vi "Dashboard Main.vi"() -> ()   [LabVIEW 2013]
uses:
  <vilib>/Rock Robotics/SystemInterfaces/AI/FPGA_AIChannel.ctl
  <vilib>/Rock Robotics/SystemInterfaces/Typedef/FPGA_TypedefAnalogModule.ctl
  <vilib>/event_ctls.llb/eventvkey.ctl
  <vilib>/Rock Robotics/WPI/Dashboard/WPI_DashboardLogging Global.vi
  <vilib>/Utility/config.llb/Write Key (String).vi
  <vilib>/Utility/config.llb/Write Key (I32).vi
  <vilib>/Utility/config.llb/NI_LVConfig.lvlib
panel:
  out "Image Message":string="Timeout in Camera Communications"
  in  "Dashboard Tab":T1(tab)
  in  "Camera Settings":T2={"Frame Rate"=30, "Compression"=30, "Size"=1} {"Frame Rate" scale=1.0..30.0; "Size" items=["640x480", "320x240", "160x120"]}
  out "MotorSliders R":cluster{"MotorSlide1":dbl, "MotorSlide2":dbl} {"MotorSlide2" scale=-1.0..1.0 scale format="%#_2e"; "MotorSlide1" scale=-1.0..1.0 scale format="%#_2e"}
  out "MotorChart R":cluster{"Numeric":dbl, "Numeric":dbl}(graph)
  out "MotorSliders L":T3 {"MotorSlide4 2" scale=0.0..14.0 scale format="%#_2e"; "MotorSlide2" scale=-1.0..1.0 scale format="%#_2e"; "MotorSlide1" scale=-1.0..1.0 scale format="%#_2e"}
  out "MotorChart L":T4(graph)
  out "JS1 Z":dbl(slide) scale=-1.0..1.0 scale format="%#_2e"
  out "Joystick 1":cluster{"X":dbl, "Y":dbl}[](graph)
  out "JS Buttons 1":T5
  out "JS2 Z":dbl(slide) scale=-1.0..1.0 scale format="%#_2e"
  out "Joystick 2":cluster{"X":dbl, "Y":dbl}[](graph)
  out "JS Buttons 2":T5
  out "Mode":T6(ring)=enum."Auto Disabled"
  out "Camera IP":string
  in  "DB Camera Config":bool
  out "fps":dbl format="%#.1g"
  out "Mbps":dbl format="%#.1g"
  out "Mbps 2":bool
  out "LED 1":bool
  in  "Enable":bool
  in  "?":dbl(slide) scale=0.0..100.0
  in  "Rec Mode":enum32{"Stop", "Record", "Playback"}(radio)
  out "distance":dbl(slide)=125.0 scale=0.0..250.0 scale format="%3d"
  in  "Scaling factor (V/in)":dbl=0.0098
  in  "Analog Module":T7
  in  "Samples Per Second":dbl=1000.0
  in  "Average Bits":u8=3 max=15
  in  "Channel":T8
  in  "stop":bool
  in  "Slider 1":dbl(slide) scale=0.0..100.0
  in  "Checkbox 2":bool
  in  "Checkbox 1":bool
  in  "Test Slider":dbl(slide) scale=0.0..100.0 scale format="%#_3g"
  in  "On/Off":bool caption="Solenoid"
  in  "Test Name":u16(ring) items=["Select the test to run...", "Example Test", "-------------------------------", "List of tests is built in robot code.", "Replace with your own automated tests."]
  in  "Test Tree":string(tree)
  in  "Motor":cluster{"Value":dbl, "Enable":bool} {"Value" scale=-1.0..1.0 scale format="%#_3g"}
  out "Progress":T9 {"Test Progress" scale=0.0..100.0}
  in  "Rev/Fwd":cluster{"Forward":bool, "Reverse":bool}
  in  "Test Ring":u16(ring) items=["Auto", "Fixed indoor", "Fixed outdoor 1", "Fixed outdoor 2", "Fixed fluorescent 1", "Fixed fluorescent 2", "Hold current"]
  in  "Listbox":i32(listbox)
  out "Tree":string(tree)
  out "Camera Image":T10(plugin-control)
  # "Left"
  # "Front"
  # "Right"
  # "Battery"
  # "Customize by placing controls and indicators here and name to\nmatch Dashboard Variables on robot."
  # "These can be set while running."
  # "Set these inputs before running."
  # "Output information."
  # "EZ1"
  # "inches"
  # "This tab is a great place for autonomous settings and validation.\nCustomize by placing controls and indicators here and name to\nmatch Dashboard Variables on robot."
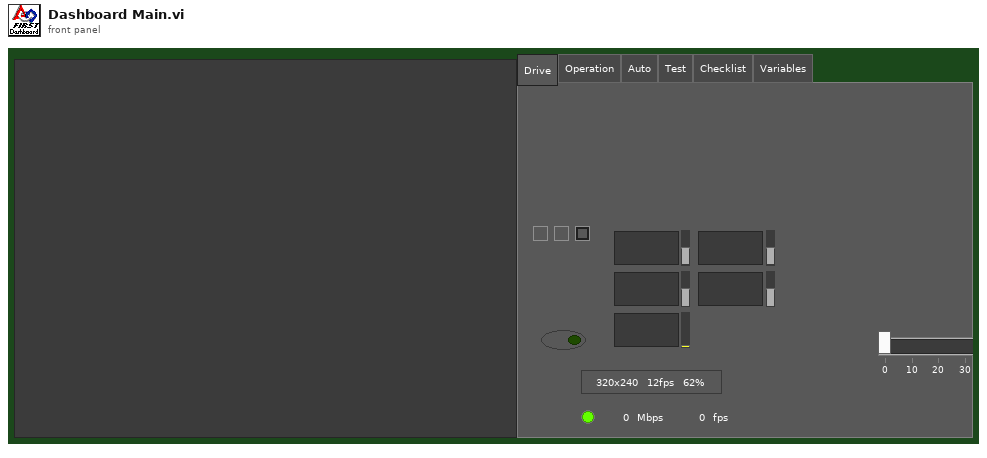
[diagram p1: front panel]
types:
  T1 = enum32{"Drive", "Operation", "Auto", "Test", "Checklist", "Variables"}
  T2 = cluster{"Frame Rate":i32, "Compression":i32, "Size":u16}
  T3 = cluster{"MotorSlide1":dbl, "MotorSlide2":dbl, "MotorSlide4 2":dbl}
  T4 = cluster{"Numeric":dbl, "Numeric":dbl, "Battery":sgl}
  T5 = cluster{bool, bool, bool, bool, bool, bool, bool, bool, bool, bool, bool, bool}
  T6 = enum8{"Tele-Op Disabled", "Tele-Op Enabled", "Auto Disabled", "Auto Enabled", "Test Disabled", "Test Enabled", ""}
  T7 = typedef "FPGA_TypedefAnalogModule.ctl" = enum16{"Analog Module 1", "Analog Module 2"}
  T8 = typedef "FPGA_AIChannel.ctl" = enum8{"AI 1", "AI 2", "AI 3", "AI 4", "AI 5", "AI 6", "AI 7", "AI 8", "Invalid"}
  T9 = cluster{"Test Progress":u8, "Test Progress Text":string}
  T10 = typedef "IMAQ Image.ctl" = refnum<image>
  T11 = typedef "Image Type" = u32
  T12 = cluster{"Digital Inputs":bool[], "Digital Outputs":bool[]}
  T13 = cluster{"Competition mode":bool, "Robot Link":bool, "Autonomous":bool, "Enabled":bool, "E-Stop":bool, "Simulated":bool, "TestMode":bool, "Docked Window":bool}
  T14 = cluster{"Boolean Array[0]":bool, "Boolean Array[1]":bool, "Boolean Array[2]":bool, "Boolean Array[3]":bool, "Boolean Array[4]":bool, "Boolean Array[5]":bool, "Boolean Array[6]":bool, "Boolean Array[7]":bool, "Boolean Array[8]":bool, "Boolean Array[9]":bool, "Boolean Array[10]":bool, "Boolean Array[11]":bool}
  T15 = typedef "NI_LVConfig.lvlib/Config Data RefNum.ctl" = refnum<k1>
  T16 = typedef "eventvkey.ctl" = enum16{"ASCII", "Enter", "Return", "Shift", "Ctrl", "Alt", "Cmd", "Opt", "Caps", "NumLock", "Clear", "Break", "Up", "Down", "Left", "Right", "Insert", "Delete", "Home", "End", "PageUp", "PageDown", "Escape", "Help", "Pause", "ScrollLock", "F1", "F2", "F3", "F4", "F5", "F6", "F7", "F8", "F9", "F10", "F11", "F12", "F13", "F14", "F15", "F16", "F17", "F18", "F19", "F20", "F21", "F22", "F23", "F24", "Play", "VolumeUp", "VolumeDown", "Mute", "Two Byte Char"}
  T17 = cluster{"Image Size":bool, "Image Type":bool, "Pixel Value":bool, "ROI Information":bool, "Zoom Factor":bool}
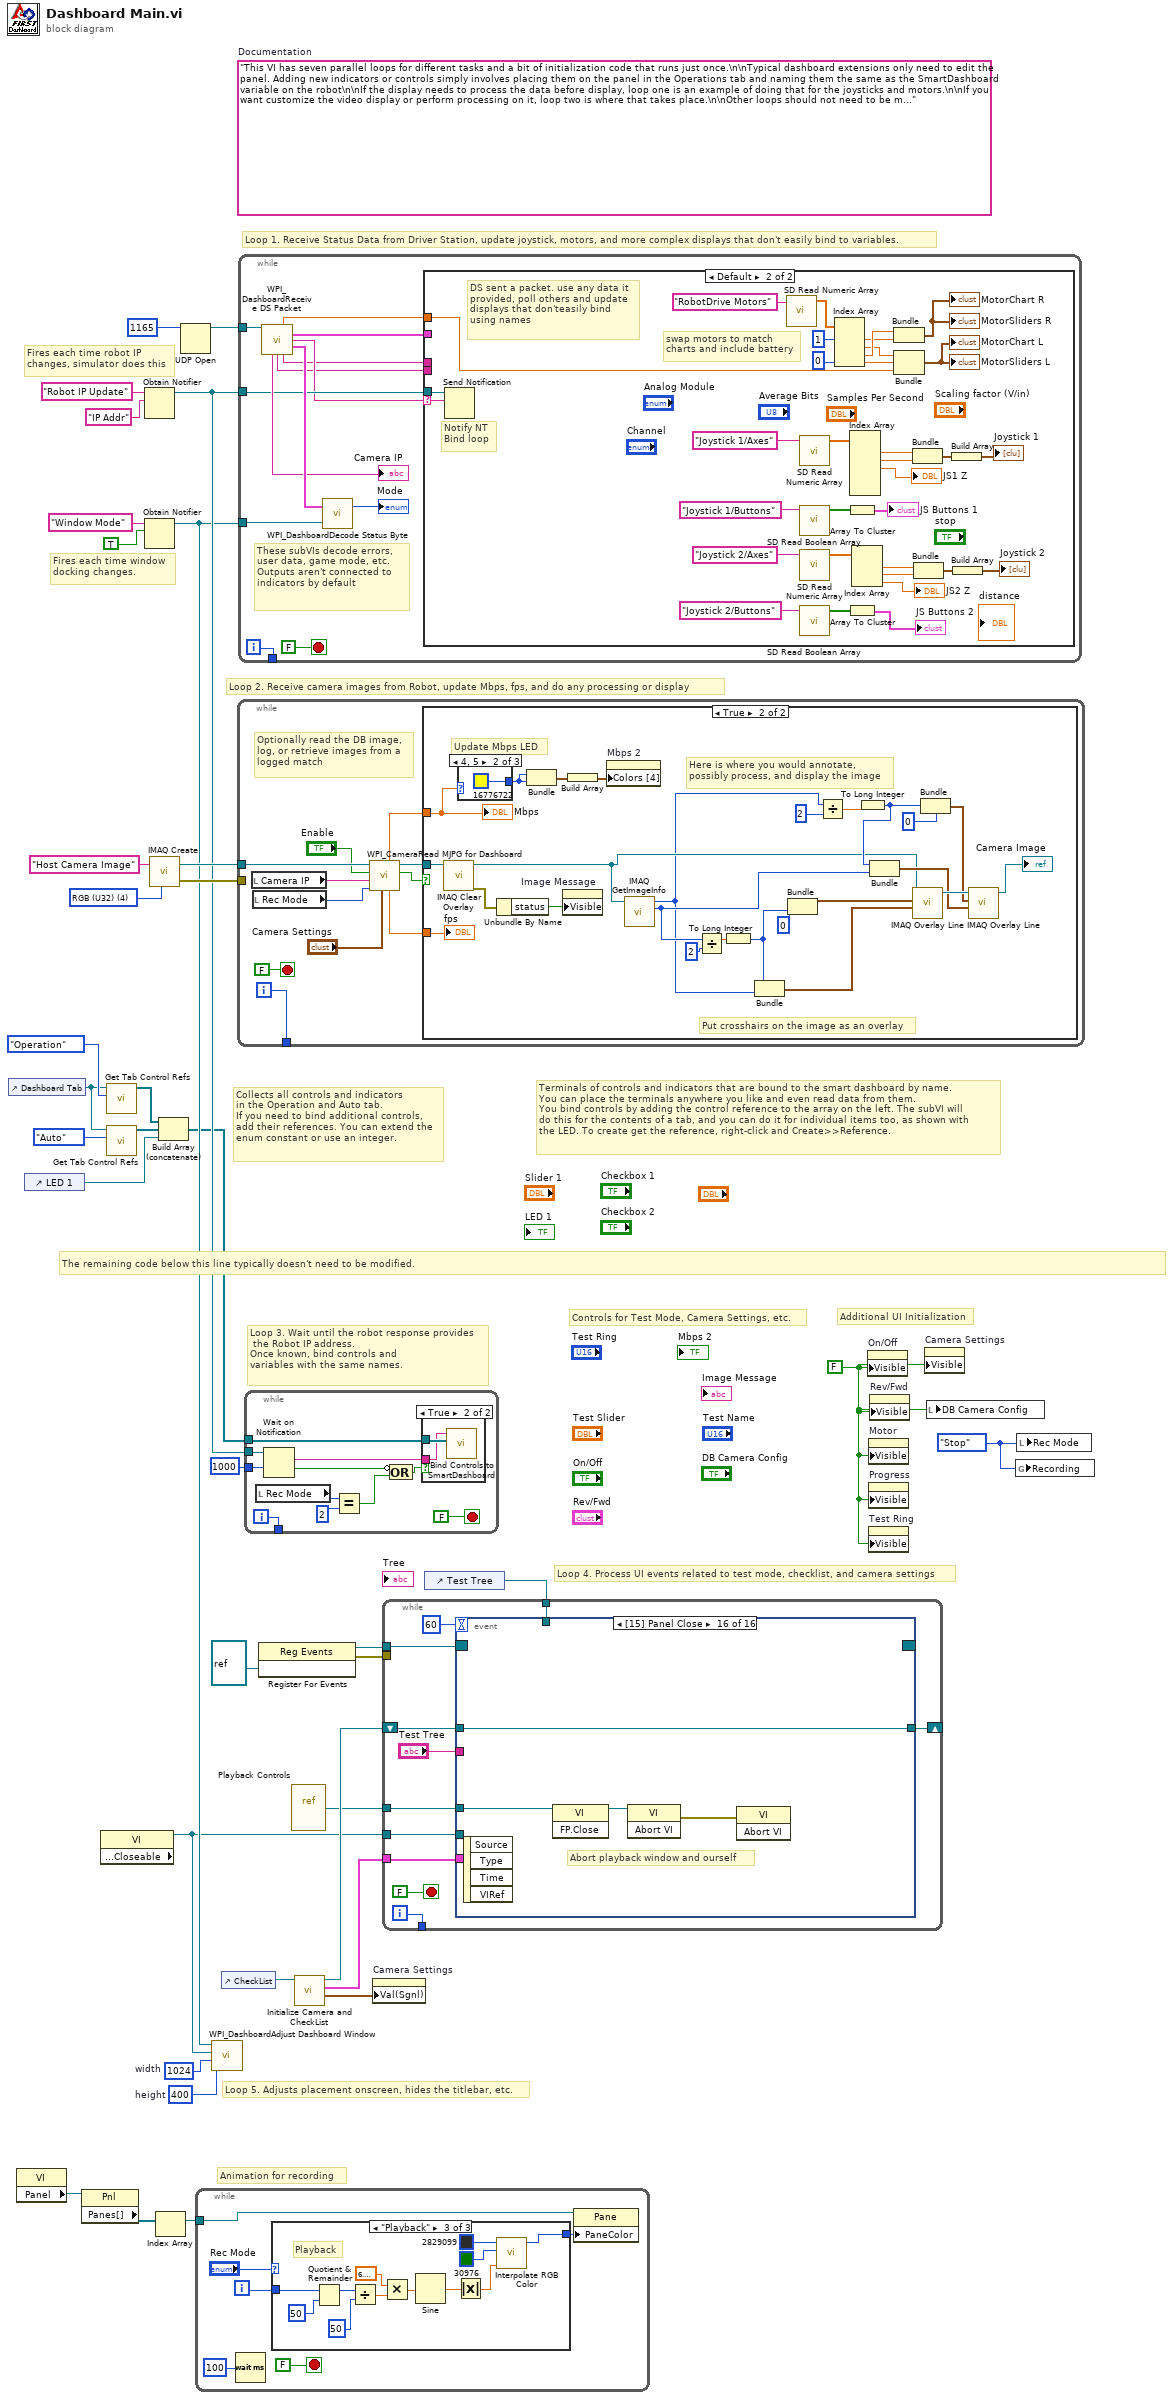
[diagram p0: block diagram]
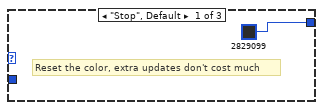
[diagram p2: hidden frame]
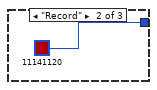
[diagram p3: hidden frame]
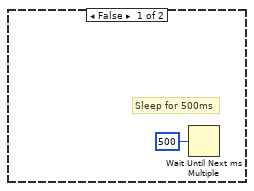
[diagram p5: hidden frame]
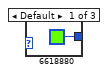
[diagram p6: hidden frame]
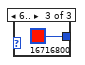
[diagram p7: hidden frame]
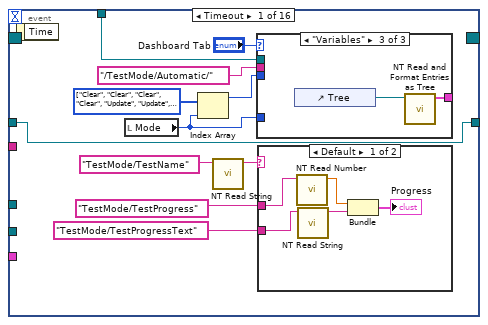
[diagram p8: hidden frame]
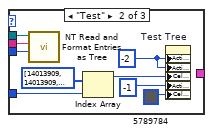
[diagram p10: hidden frame]
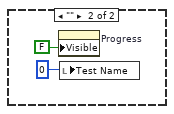
[diagram p11: hidden frame]
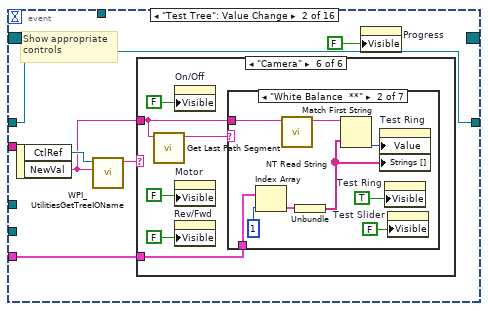
[diagram p12: hidden frame]
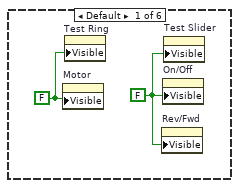
[diagram p13: hidden frame]
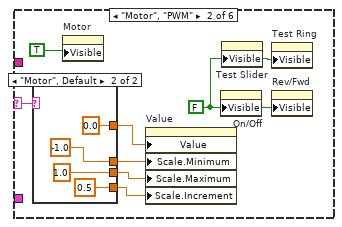
[diagram p14: hidden frame]
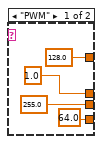
[diagram p15: hidden frame]
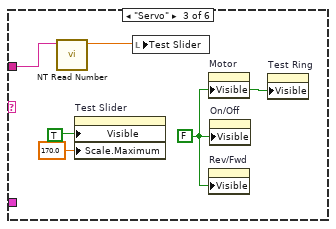
[diagram p16: hidden frame]
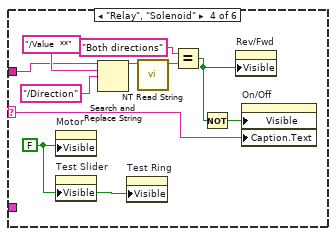
[diagram p17: hidden frame]
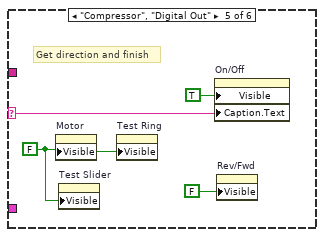
[diagram p18: hidden frame]
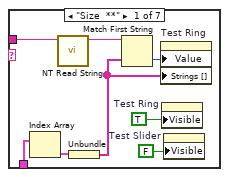
[diagram p19: hidden frame]
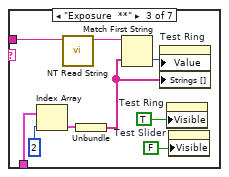
[diagram p20: hidden frame]
diagram:
  w8 = enum32{"Stop", "Record", "Playback"}."Stop" ("Rec Mode")
  w11 = 400  # height
  w12 = 1024  # width
  w25 = FALSE ("Visible")
  (unwired) "This VI has seven parallel loops for different tasks and a bit of initialization code that runs just once.\n\nTypical dashboard extensions only need to edit the panel. Adding new indicators or controls simply involves placing them on the panel in the Operations tab and naming them the same as the SmartDashboard variable on the robot\n\nIf the display needs to process the data before display, loop one is an example of doing that for the joysticks and motors.\n\nIf you want customize the video display or perform processing on it, loop two is where that takes place.\n\nOther loops should not need to be modified. They are pretty standard, and document the task they perform."  # Documentation
  w35 = T11 4 items=["Grayscale (U8)", "Grayscale (I16)", "Grayscale (SGL)", "Complex (CSG)", "RGB (U32)", "HSL (U32)", "RGB (U64)"] ("Image Type")
  # "Controls for Test Mode, Camera Settings, etc."
  # "Additional UI Initialization"
  # "Animation for recording"
  # "Fires each time robot IP\nchanges, simulator does this"
  # "Fires each time window\ndocking changes."
  # "Collects all controls and indicators\nin the Operation and Auto tab.\nIf you need to bind additional controls,\nadd their references. You can extend the\nenum constant or use an integer."
  # "The remaining code below this line typically doesn't need to be modified."
  # "Loop 4. Process UI events related to test mode, checklist, and camera settings"
  # "Terminals of controls and indicators that are bound to the smart dashboard by name.\nYou can place the terminals anywhere you like and even read data from them.\nYou bind controls by adding the control reference to the array on the left. The subVI will\ndo this for the contents of a tab, and you can do it for individual items too, as shown with\nthe LED. To create get the reference, right-click and Create>>Reference."
  # "Loop 3. Wait until the robot response provides\n the Robot IP address.\nOnce known, bind controls and\nvariables with the same names."
  # "Loop 5. Adjusts placement onscreen, hides the titlebar, etc."
  # "Loop 1. Receive Status Data from Driver Station, update joystick, motors, and more complex displays that don't easily bind to variables."
  # "Loop 2. Receive camera images from Robot, update Mbps, fps, and do any processing or display"
  n1 = control-ref of="Dashboard Tab"() -> (w6:refnum<vi>)
  n2 = property class="VI"() -> ("Panel"=w19:refnum<vi>)  [unwired: 2 in, 2 out]
  n3 = control-ref of="LED 1"() -> (w1:refnum<vi>)
  n4 = property class="Pnl"(reference=w19) -> ("Panes[]"=w20:refnum<vi>[])  [unwired: 1 in, 2 out]
  n5 = property class="VI" props=["Front Panel.Closeable"]() -> (reference out=w7:refnum<vi>)  [unwired: 2 in, 2 out]
  n6 = call <vilib>:"Get Tab Control Refs.vi"("Page Index"=T1."Operation" ("Dashboard Tab"), "TabControl in"=w6) -> ("ControlsOnPage"=w4:refnum<vi>[])  [unwired: 9 in]
  n7 = call <vilib>:"Get Tab Control Refs.vi"("Page Index"=T1."Auto" ("Dashboard Tab"), "TabControl in"=w6) -> ("ControlsOnPage"=w5:refnum<vi>[])  [unwired: 9 in]
  n8 = Obtain Notifier(name (unnamed)="Robot IP Update", notification data type="IP Addr" ("name (unnamed)")) -> (notifier out=w29:refnum<notifier>)  [unwired: 2 in, 2 out]
  n9 = Obtain Notifier(name (unnamed)="Window Mode", notification data type=TRUE) -> (notifier out=w10:refnum<notifier>)  [unwired: 2 in, 2 out]
  n10 = call "IMAQ Create"("Image Name"="Host Camera Image", "Image Type"=w35) -> ("New Image"=w33:T10, "error out"=w32:errorcluster)  [unwired: 2 in, 1 out]
  n11 = Index Array(array=w20) -> (element=w18:refnum<vi>)  [unwired: 1 in]
  n12 = Build Array (concatenate)(w4, w5, w1) -> (w3:refnum<vi>[])
  n13 = UDP Open(11:u16 1165 ("port")) -> (port=w36:refnum<k16>)  [unwired: 2 in, 4 out]
  n14 = while {
    tunnel: w18 -> [w39]
    i -> [w42]
    stop <- FALSE stop-if-true
    n15 = Wait (ms)(milliseconds to wait=u32 100) -> ()  [unwired: 1 out]
    n16 = case shown="\"Playback\"" "Rec Mode" {
      tunnel: w42 -> [_ _ w57]
      tunnel: [u32 2829099 ("Base Color") u32 11141120 ("Target Color") w46] -> w38
      frame "Stop", Default {
        # "Reset the color, extra updates don't cost much"
      }
      frame "Record" {
      }
      frame "Playback" {
        # "Playback"
        n17 = Quotient & Remainder(x=w57, y=u32 50 ("milliseconds to wait")) -> (x-y*floor(x/y)=w53:u32)  [unwired: 1 out]
        n18 = Divide(x=w53, y=u32 50 ("milliseconds to wait")) -> (x/y=w50:dbl)
        n19 = Multiply(x=6.283185307179586, y=w50) -> (x*y=w55:dbl)
        n20 = Sine(x=w55) -> (sin(x)=w54:dbl)
        n21 = Absolute Value(x=w54) -> (abs(x)=w47:dbl)
        n22 = call "Interpolate RGB Color.vi"("Proportion"=w47, "Target Color"=u32 30976, "Base Color"=u32 2829099) -> ("Result Color"=w46:u32)  [unwired: 8 in]
      }
    }
    n23 = property class="Pane"(reference=w39, "PaneColor"=w38) -> ()  [unwired: 1 in, 2 out]
  }
  n24 = call <vilib>:"WPI_DashboardAdjust Dashboard Window.vi"("height"=w11, "width"=w12, "reference in"=w7, "Notifier in"=w10) -> ()  [unwired: 8 in]
  n25 = control-ref of="CheckList"() -> (w9:refnum<vi>)
  n26 = while {
    tunnel: w33 -> [w66]
    tunnel: w32 -> [_]
    tunnel: [w67] -> _
    i -> [w67]
    stop <- FALSE stop-if-true
    # "Optionally read the DB image,\nlog, or retrieve images from a\nlogged match"
    n27 = local read "Camera IP"() -> (w59:string)
    n28 = local read "Rec Mode"() -> (w58:enum32{"Stop", "Record", "Playback"})
    n29 = call <vilib>:"WPI_CameraRead MJPG for Dashboard.vi"("Camera Settings"="Camera Settings", "Rec Mode"=w58, "Camera IP"=w59, "Enable"="Enable", "Refnum in"=w66) -> ("Active"=w63:bool, "Refnum out"=w65:T10, "FPS"=w62:dbl, "Bandwidth (Mbps)"=w61:dbl)  [unwired: 3 in]
    n30 = case shown="True" w63 {
      tunnel: w65 -> [_ w89]
      tunnel: w61 -> [_ w88]
      tunnel: w62 -> [_ w87]
      frame False {
        # "Sleep for 500ms"
        n31 = Wait Until Next ms Multiple(millisecond multiple=u32 500) -> ()  [unwired: 1 out]
      }
      frame True {
        # "Put crosshairs on the image as an overlay"
        # "Here is where you would annotate,\npossibly process, and display the image"
        # "Update Mbps LED"
        n32 = call "IMAQ Clear Overlay"("Image"=w89) -> ("error out"=w93:errorcluster, "Image Out"=w72:T10)  [unwired: 2 in, 7 out]
        n33 = case shown="4, 5" w88 {
          tunnel: [u32 6618880 ("Color Box") u32 16776722 ("Color Box") u32 16716800 ("Color Box")] -> w90
          frame Default {
          }
          frame 4, 5 {
          }
          frame 6.. {
          }
        }
        n34 = Unbundle By Name(w93) -> ("status"=w94:bool)
        n35 = Bundle("Color Box"=w90, "Color Box"=w90) -> (w92:cluster{"Color Box":u32, "Color Box":u32})  [unwired: 1 out]
        n36 = property on="Image Message" class="Str"("Visible"=w94) -> ()  [unwired: 2 in, 2 out]
        n37 = Build Array(w92) -> (w91:cluster{"Color Box":u32, "Color Box":u32}[])
        n38 = property on="Mbps 2" class="Bool (strict)"("Colors [4]"=w91) -> ()  [unwired: 2 in, 2 out]
        n39 = call "IMAQ GetImageInfo"("Image"=w72) -> ("Y Resolution"=w76:i32, "X Resolution"=w70:i32)  [unwired: 3 in, 6 out]
        n40 = Divide(x=w76, y=2) -> (x/y=w81:dbl)
        n41 = To Long Integer(number=w81) -> (32bit integer=w78:i32)
        n42 = Bundle(w78, "X Resolution"=w70) -> (w77:cluster{i32, "X Resolution":i32})  [unwired: 1 in]
        n43 = Bundle(0, w78) -> (w80:cluster{i32, i32})  [unwired: 1 in]
        n44 = Divide(x=w70, y=2) -> (x/y=w85:dbl)
        n45 = To Long Integer(number=w85) -> (32bit integer=w74:i32)
        n46 = Bundle(w74, "Y Resolution"=w76) -> (w75:cluster{i32, "Y Resolution":i32})  [unwired: 1 in]
        n47 = call "IMAQ Overlay Line"("End Point"=w77, "Start Point"=w80, "Image"=w72) -> ("Image Out"=w83:T10)  [unwired: 7 in, 1 out]
        n48 = Bundle(w74, 0) -> (w73:cluster{i32, i32})  [unwired: 1 in]
        n49 = call "IMAQ Overlay Line"("End Point"=w75, "Start Point"=w73, "Image"=w83) -> ("Image Out"=→"Camera Image":T10)  [unwired: 7 in, 1 out]
        "Mbps" <- w88
        "fps" <- w87
      }
    }
  }
  n50 = while {
    tunnel: w36 -> [w108]
    tunnel: w29 -> [w103]
    tunnel: w10 -> [w107]
    tunnel: [w104] -> _
    i -> [w104]
    stop <- FALSE stop-if-true
    # "These subVIs decode errors, user data, game mode, etc.\nOutputs aren't connected to indicators by default"
    n51 = call <vilib>:"WPI_DashboardReceive DS Packet.vi"("Recv Socket"=w108) -> ("Battery"=w98:sgl, "Driver Station"=w99:T12, "Robot IP Address"=w102:string, "Status"=w109:T13, "Camera IP Address"=→"Camera IP":string, "Low Priority User Data"=w101:string, "High Priority User Data"=w100:string)  [unwired: 1 in, 7 out]
    n52 = call <vilib>:"WPI_DashboardDecode Status Byte.vi"("Window Mode Notifier"=w107, "Status"=w109) -> ("Mode"=→"Mode":T6)  [unwired: 1 out]
    n53 = case shown="Default" w102 {
      selector: w102 -> [_ w121]
      tunnel: w103 -> [_ w122]
      tunnel: w101 -> [_ _]
      tunnel: w100 -> [_ _]
      tunnel: w99 -> [_ _]
      tunnel: w98 -> [_ w120]
      frame "0.0.0.0" {
        # "DS not sending packets, or no robot exists yet.\nDon't poll the variables"
      }
      frame Default {
        # "Notify NT\nBind loop"
        # "DS sent a packet. use any data it\nprovided, poll others and update\ndisplays that don'teasily bind\nusing names"
        # "swap motors to match\ncharts and include battery"
        n54 = Send Notification(notification=w121, notifier=w122) -> ()  [unwired: 1 in, 2 out]
        n55 = call <vilib>:"SD Read Numeric Array.vi"("Name"="RobotDrive Motors") -> ("Numeric Array"=w119:dbl[])  [unwired: 8 in, 2 out]
        n56 = call <vilib>:"SD Read Numeric Array.vi"("Name"="Joystick 1/Axes") -> ("Numeric Array"=w138:dbl[])  [unwired: 8 in, 2 out]
        n57 = call <vilib>:"SD Read Boolean Array.vi"("Name"="Joystick 1/Buttons") -> ("Boolean Array"=w140:bool[])  [unwired: 8 in, 2 out]
        n58 = call <vilib>:"SD Read Numeric Array.vi"("Name"="Joystick 2/Axes") -> ("Numeric Array"=w132:dbl[])  [unwired: 8 in, 2 out]
        n59 = call <vilib>:"SD Read Boolean Array.vi"("Name"="Joystick 2/Buttons") -> ("Boolean Array"=w131:bool[])  [unwired: 8 in, 2 out]
        n60 = Index Array(array=w119, index #1=1, index #4=0) -> (element #1=w115:dbl, element #2=w114:dbl, element #3=w116:dbl, element #4=w111:dbl)  [unwired: 2 in]
        n61 = Array To Cluster(array=w140) -> (cluster=→"JS Buttons 1":T14)
        n62 = Array To Cluster(array=w131) -> (cluster=→"JS Buttons 2":T14)
        n63 = Index Array(array=w138) -> (element #1=w135:dbl, element #2=w136:dbl, element #3=→"JS1 Z":dbl)  [unwired: 6 in, 3 out]
        n64 = Index Array(array=w132) -> (element #1=w127:dbl, element #2=w126:dbl, element #3=→"JS2 Z":dbl)  [unwired: 3 in]
        n65 = Bundle("Numeric"=w116, "Numeric"=w115) -> (→"MotorChart R" →"MotorSliders R":cluster{"Numeric":dbl, "Numeric":dbl})  [unwired: 1 in]
        n66 = Bundle("Numeric"=w114, "Numeric"=w111, "Battery"=w120) -> (→"MotorChart L" →"MotorSliders L":T4)  [unwired: 1 in]
        n67 = Bundle("Numeric"=w135, "Numeric"=w136) -> (w134:cluster{"Numeric":dbl, "Numeric":dbl})  [unwired: 1 in]
        n68 = Bundle("Numeric"=w127, "Numeric"=w126) -> (w128:cluster{"Numeric":dbl, "Numeric":dbl})  [unwired: 1 in]
        n69 = Build Array(w134) -> (→"Joystick 1":cluster{"Numeric":dbl, "Numeric":dbl}[])
        n70 = Build Array(w128) -> (→"Joystick 2":cluster{"Numeric":dbl, "Numeric":dbl}[])
      }
    }
  }
  n71 = while {
    tunnel: w3 -> [w154]
    tunnel: w29 -> [w152]
    tunnel: [w150] -> _
    tunnel: u32 1000 ("milliseconds to wait") -> [w149]
    i -> [w150]
    stop <- FALSE stop-if-true
    n72 = local read "Rec Mode"() -> (w145:enum32{"Stop", "Record", "Playback"})
    n73 = Wait on Notification(notifier=w152, timeout in ms (-1)=w149) -> (notification=w151:string, timed out?=w147:bool)  [unwired: 2 in, 2 out]
    n74 = Equal?(x=w145, y=u16 2 ("Rec Mode")) -> (x = y?=w146:bool)
    n75 = Compound Arithmetic op=OR(invert w147, w146) -> (w148:bool)
    n76 = case shown="True" w148 {
      tunnel: w154 -> [_ w156]
      tunnel: w151 -> [_ w155]
      frame False {
      }
      frame True {
        n77 = call <vilib>:"Bind Controls to SmartDashboard.vi"("Bound Control Refs"=w156, "Server IP Address"=w155) -> ()  [unwired: 10 in]
      }
    }
  }
  n78 = register-events(refnum<vi> refnum) -> (reference out=w16:refnum<event-registration>, error out=w15:errorcluster)  [unwired: 2 in]
  n79 = vi-ref "Playback Controls.vi"() -> (w17:refnum<vi>)
  n80 = call "Initialize Camera and CheckList.vi"("ListBox in"=w9) -> ("Cluster"=w23:cluster{"value":i32, "value":i32, "index":i32}, "Array"=w24:cluster{string[]}[], "File Refnum"=w22:T15)  [unwired: 8 in]
  n81 = property on="Camera Settings" class="Clust (strict)"("Val(Sgnl)"=w23) -> ()  [unwired: 2 in, 2 out]
  n82 = control-ref of="Test Tree"() -> (w21:refnum<vi>)
  n83 = while {
    tunnel: w24 -> [w164]
    shift-right: [w163] -> _
    shift-left: w22 -> [w162]
    tunnel: [w161] -> _
    tunnel: w21 -> [w160]
    tunnel: w17 -> [w159]
    tunnel: w16 -> [w158]
    tunnel: w15 -> [_]
    tunnel: w7 -> [w157]
    i -> [w161]
    stop <- FALSE stop-if-true
    n84 = event shown="[15] Panel Close" {
      selector: w158 -> [_ _ _ _ _ _ _ _ _ _ _ _ _ _ _ _]
      dyn-events: [_ _ _ _ _ _ _ _ _ _ _ _ _ w402 _ _] -> _
      timeout: u32 60 ("milliseconds to wait") -> [_ _ _ _ _ _ _ _ _ _ _ _ _ _ _ _]
      tunnel: w160 -> [w174 _ _ _ _ _ _ _ _ _ _ _ _ _ _ _]
      tunnel: "Test Tree" -> [_ _ _ _ _ _ _ _ w371 w379 w381 w385 w393 _ _ _]
      tunnel: w164 -> [_ w198 _ _ _ _ w335 w365 _ _ _ _ _ _ _ _]
      tunnel: [w168 w197 w296 w301 w309 w321 w334 w358 w370 w377 w380 w384 w392 w404 w418 w419] -> w163
      tunnel: w162 -> [w168 w197 w296 w301 w309 w321 w333 w358 w370 w377 w380 w384 w392 w404 w418 w419]
      tunnel: w159 -> [_ _ _ _ _ _ _ _ _ _ _ _ _ w405 _ w422]
      tunnel: w157 -> [_ _ _ _ _ _ _ _ _ _ _ _ _ w400 _ _]
      event Timeout {
        w173 = enum16{"Update", "Clear"}[] [enum."Clear", enum."Clear", enum."Clear", enum."Clear", enum."Update", enum."Update", enum."Clear"] items=["Update", "Clear"]
        n85 = event-data() -> ()  [unwired: 1 in, 1 out]
        n86 = local read "Mode"() -> (w171:T6)
        n87 = Index Array(array=w173, index=w171) -> (element=w172:enum16{"Update", "Clear"})
        n88 = call <vilib>:"NT Read String.vi"("Name"="TestMode/TestName") -> ("String"=w177:string)  [unwired: 9 in, 1 out]
        n89 = case shown="\"Variables\"" "Dashboard Tab" {
          tunnel: w174 -> [_ w187 _]
          tunnel: "/TestMode/Automatic/" ("Name Pattern") -> [_ w186 _]
          tunnel: w172 -> [_ w185 _]
          tunnel: w171 -> [_ w183 _]
          tunnel: [_ _ w189] -> _
          frame "Operation", Default {
          }
          frame "Test" {
            w182 = -2 ("Active Item:Row Number")
            n90 = call <vilib>:"NT Read and Format Entries as Tree.vi"("Operation"=w185, "Name Pattern"=w186, "Tree Refnum"=w187) -> ()  [unwired: 7 in, 2 out]
            n91 = Index Array(array=u32[] [14013909, 14013909, 14013909, 14013909, 14013909, 16777215, 14013909], index=w183) -> (element=w181:u32)
            n92 = property on="Test Tree" class="Tree (strict)"("Active Item Row Number"=w182, "ActiveColNum"=w182, "CellBG"=w181, "Active Item Row Number"=-1 ("Active Item:Row Number"), "CellBG"=u32 5789784 ("Color Box")) -> ()  [unwired: 2 in, 2 out]
          }
          frame "Variables" {
            n93 = control-ref of="Tree"() -> (w188:refnum<vi>)
            n94 = call <vilib>:"NT Read and Format Entries as Tree.vi"("Tree Refnum"=w188) -> ("Formatted Strings"=w189:cluster{"Name":string, "Value":string}[])  [unwired: 9 in, 1 out]
          }
        }
        n95 = case shown="Default" w177 {
          tunnel: "TestMode/TestProgress" ("Name") -> [w191 _]
          tunnel: "TestMode/TestProgressText" ("Name") -> [w190 _]
          frame Default {
            n96 = call <vilib>:"NT Read Number.vi"("Name"=w191) -> ("Numeric"=w192:dbl)  [unwired: 9 in, 1 out]
            n97 = call <vilib>:"NT Read String.vi"("Name"=w190) -> ("String"=w193:string)  [unwired: 9 in, 1 out]
            n98 = Bundle("Numeric"=w192, "String"=w193) -> (→"Progress":cluster{"Numeric":dbl, "String":string})  [unwired: 1 in]
          }
          frame "" {
            n99 = property on="Progress" class="Clust (strict)"("Visible"=FALSE) -> ()  [unwired: 2 in, 2 out]
            n100 = local write "Test Name"(u16 0) -> ()
          }
        }
      }
      event "Test Tree": Value Change {
        # "Show appropriate\ncontrols"
        n101 = event-data() -> ("CtlRef"=w201:refnum<vi>, "NewVal"=w199:string)  [unwired: 1 in]
        n102 = call <vilib>:"WPI_UtilitiesGetTreeIOName.vi"("NewVal"=w199, "TreeControl in"=w201) -> ("I/O Name"=w202:string)  [unwired: 9 in]
        n103 = case shown="\"Camera\"" w202 {
          selector: w202 -> [_ w209 _ w227 w236 _]
          tunnel: w199 -> [_ _ w224 w226 _ w243]
          tunnel: w198 -> [_ _ _ _ _ w242]
          frame Default {
            w204 = FALSE ("Visible")
            w203 = FALSE ("Visible")
            n104 = property on="Motor" class="Clust (strict)"("Visible"=w203) -> ()  [unwired: 2 in, 2 out]
            n105 = property on="Test Ring" class="Ring (strict)"("Visible"=w203) -> ()  [unwired: 2 in, 2 out]
            n106 = property on="Rev/Fwd" class="Clust (strict)"("Visible"=w204) -> ()  [unwired: 2 in, 2 out]
            n107 = property on="On/Off" class="Bool (strict)"("Visible"=w204) -> ()  [unwired: 2 in, 2 out]
            n108 = property on="Test Slider" class="Slide (strict)"("Visible"=w204) -> ()  [unwired: 2 in, 2 out]
          }
          frame "Motor", "PWM" {
            w210 = FALSE ("Visible")
            n109 = case shown="\"Motor\", Default" w209 {
              tunnel: [1.0 ("Value") -1.0 ("Value")] -> w208
              tunnel: [255.0 ("Value") 1.0 ("Value")] -> w207
              tunnel: [128.0 ("Value") 0.0 ("Value")] -> w206
              tunnel: [64.0 ("Value") 0.5 ("Value")] -> w205
              frame "PWM" {
              }
              frame "Motor", Default {
              }
            }
            n110 = property on="Motor" class="Clust (strict)"("Visible"=TRUE) -> ()  [unwired: 2 in, 2 out]
            n111 = property on="Value" class="Slide (strict)"("Value"=w206, "Scale.Minimum"=w208, "Scale.Maximum"=w207, "Scale.Increment"=w205) -> ()  [unwired: 2 in, 2 out]
            n112 = property on="On/Off" class="Bool (strict)"("Visible"=w210) -> ()  [unwired: 2 in, 2 out]
            n113 = property on="Test Slider" class="Slide (strict)"("Visible"=w210) -> ()  [unwired: 2 in, 2 out]
            n114 = property on="Test Ring" class="Ring (strict)"("Visible"=w210) -> ()  [unwired: 2 in, 2 out]
            n115 = property on="Rev/Fwd" class="Clust (strict)"("Visible"=w210) -> ()  [unwired: 2 in, 2 out]
          }
          frame "Servo" {
            w222 = FALSE ("Visible")
            n116 = call <vilib>:"NT Read Number.vi"("Name"=w224) -> ("Numeric"=w223:dbl)  [unwired: 9 in, 1 out]
            n117 = property on="Test Slider" class="Slide (strict)"("Visible"=TRUE, "Scale.Maximum"=170.0 ("Scale.Range:Maximum")) -> ()  [unwired: 2 in, 2 out]
            n118 = local write "Test Slider"(w223) -> ()
            n119 = property on="Motor" class="Clust (strict)"("Visible"=w222) -> ()  [unwired: 2 in, 2 out]
            n120 = property on="Rev/Fwd" class="Clust (strict)"("Visible"=w222) -> ()  [unwired: 2 in, 2 out]
            n121 = property on="On/Off" class="Bool (strict)"("Visible"=w222) -> ()  [unwired: 2 in, 2 out]
            n122 = property on="Test Ring" class="Ring (strict)"("Visible"=w222) -> ()  [unwired: 2 in, 2 out]
          }
          frame "Relay", "Solenoid" {
            w225 = FALSE ("Visible")
            n123 = property on="Motor" class="Clust (strict)"("Visible"=w225) -> ()  [unwired: 2 in, 2 out]
            n124 = property on="Test Slider" class="Slide (strict)"("Visible"=w225) -> ()  [unwired: 2 in, 2 out]
            n125 = Search and Replace String(input string=w226, search string="/Value  **", replace string="/Direction") -> (result string=w232:string)  [unwired: 5 in, 3 out]
            n126 = property on="Test Ring" class="Ring (strict)"("Visible"=w225) -> ()  [unwired: 2 in, 2 out]
            n127 = call <vilib>:"NT Read String.vi"("Name"=w232) -> ("String"=w230:string)  [unwired: 9 in, 1 out]
            n128 = Equal?(x="Both directions", y=w230) -> (x = y?=w228:bool)
            n129 = Not(x=w228) -> (.not. x?=w229:bool)
            n130 = property on="Rev/Fwd" class="Clust (strict)"("Visible"=w228) -> ()  [unwired: 2 in, 2 out]
            n131 = property on="On/Off" class="Bool (strict)"("Visible"=w229, "Caption.Text"=w227) -> ()  [unwired: 2 in, 2 out]
          }
          frame "Compressor", "Digital Out" {
            w235 = FALSE ("Visible")
            # "Get direction and finish"
            n132 = property on="Motor" class="Clust (strict)"("Visible"=w235) -> ()  [unwired: 2 in, 2 out]
            n133 = property on="Test Slider" class="Slide (strict)"("Visible"=w235) -> ()  [unwired: 2 in, 2 out]
            n134 = property on="Test Ring" class="Ring (strict)"("Visible"=w235) -> ()  [unwired: 2 in, 2 out]
            n135 = property on="On/Off" class="Bool (strict)"("Visible"=TRUE, "Caption.Text"=w236) -> ()  [unwired: 2 in, 2 out]
            n136 = property on="Rev/Fwd" class="Clust (strict)"("Visible"=FALSE) -> ()  [unwired: 2 in, 2 out]
          }
          frame "Camera" {
            n137 = call <vilib>:"Get Last Path Segment.vi"("String in"=w243) -> ("String out"=w244:string)  [unwired: 10 in]
            n138 = property on="On/Off" class="Bool (strict)"("Visible"=FALSE) -> ()  [unwired: 2 in, 2 out]
            n139 = property on="Motor" class="Clust (strict)"("Visible"=FALSE) -> ()  [unwired: 2 in, 2 out]
            n140 = property on="Rev/Fwd" class="Clust (strict)"("Visible"=FALSE) -> ()  [unwired: 2 in, 2 out]
            n141 = case shown="\"White Balance  **\"" w244 {
              tunnel: w243 -> [w250 w259 w268 w277 w286 _ w292]
              tunnel: w242 -> [w248 w256 w265 w274 w283 _ _]
              frame "Size  **" {
                n142 = Index Array(array=w248) -> (element=w247:cluster{string[]})  [unwired: 1 in]
                n143 = call <vilib>:"NT Read String.vi"("Name"=w250) -> ("String"=w249:string)  [unwired: 9 in, 1 out]
                n144 = Unbundle(w247) -> (w245:string[])
                n145 = Match First String(2:w245, 3:w249) -> (0:w246:i32)  [unwired: 1 out]
                n146 = property on="Test Ring" class="Ring (strict)"("Value"=w246, "Strings []"=w245) -> ()  [unwired: 2 in, 2 out]
                n147 = property on="Test Ring" class="Ring (strict)"("Visible"=TRUE) -> ()  [unwired: 2 in, 2 out]
                n148 = property on="Test Slider" class="Slide (strict)"("Visible"=FALSE) -> ()  [unwired: 2 in, 2 out]
              }
              frame "White Balance  **" {
                n149 = Index Array(array=w256, index=1) -> (element=w257:cluster{string[]})
                n150 = call <vilib>:"NT Read String.vi"("Name"=w259) -> ("String"=w258:string)  [unwired: 9 in, 1 out]
                n151 = Unbundle(w257) -> (w254:string[])
                n152 = Match First String(2:w254, 3:w258) -> (0:w253:i32)  [unwired: 1 out]
                n153 = property on="Test Ring" class="Ring (strict)"("Value"=w253, "Strings []"=w254) -> ()  [unwired: 2 in, 2 out]
                n154 = property on="Test Ring" class="Ring (strict)"("Visible"=TRUE) -> ()  [unwired: 2 in, 2 out]
                n155 = property on="Test Slider" class="Slide (strict)"("Visible"=FALSE) -> ()  [unwired: 2 in, 2 out]
              }
              frame "Exposure  **" {
                n156 = Index Array(array=w265, index=2) -> (element=w266:cluster{string[]})
                n157 = call <vilib>:"NT Read String.vi"("Name"=w268) -> ("String"=w267:string)  [unwired: 9 in, 1 out]
                n158 = Unbundle(w266) -> (w262:string[])
                n159 = Match First String(2:w262, 3:w267) -> (0:w263:i32)  [unwired: 1 out]
                n160 = property on="Test Ring" class="Ring (strict)"("Value"=w263, "Strings []"=w262) -> ()  [unwired: 2 in, 2 out]
                n161 = property on="Test Ring" class="Ring (strict)"("Visible"=TRUE) -> ()  [unwired: 2 in, 2 out]
                n162 = property on="Test Slider" class="Slide (strict)"("Visible"=FALSE) -> ()  [unwired: 2 in, 2 out]
              }
              frame "Exposure Priority  **" {
                n163 = Index Array(array=w274, index=3) -> (element=w275:cluster{string[]})
                n164 = call <vilib>:"NT Read String.vi"("Name"=w277) -> ("String"=w276:string)  [unwired: 9 in, 1 out]
                n165 = Unbundle(w275) -> (w271:string[])
                n166 = Match First String(2:w271, 3:w276) -> (0:w272:i32)  [unwired: 1 out]
                n167 = property on="Test Ring" class="Ring (strict)"("Value"=w272, "Strings []"=w271) -> ()  [unwired: 2 in, 2 out]
                n168 = property on="Test Ring" class="Ring (strict)"("Visible"=TRUE) -> ()  [unwired: 2 in, 2 out]
                n169 = property on="Test Slider" class="Slide (strict)"("Visible"=FALSE) -> ()  [unwired: 2 in, 2 out]
              }
              frame "Color Enable  **" {
                n170 = Index Array(array=w283, index=4) -> (element=w284:cluster{string[]})
                n171 = call <vilib>:"NT Read String.vi"("Name"=w286) -> ("String"=w285:string)  [unwired: 9 in, 1 out]
                n172 = Unbundle(w284) -> (w280:string[])
                n173 = Match First String(2:w280, 3:w285) -> (0:w281:i32)  [unwired: 1 out]
                n174 = property on="Test Ring" class="Ring (strict)"("Value"=w281, "Strings []"=w280) -> ()  [unwired: 2 in, 2 out]
                n175 = property on="Test Ring" class="Ring (strict)"("Visible"=TRUE) -> ()  [unwired: 2 in, 2 out]
                n176 = property on="Test Slider" class="Slide (strict)"("Visible"=FALSE) -> ()  [unwired: 2 in, 2 out]
              }
              frame Default {
                n177 = property on="Test Ring" class="Ring (strict)"("Visible"=FALSE) -> ()  [unwired: 2 in, 2 out]
                n178 = property on="Test Slider" class="Slide (strict)"("Visible"=FALSE) -> ()  [unwired: 2 in, 2 out]
              }
              frame "Brightness  **", "Color Level  **", "Compression  **", "FPS  **", "Sharpness  **" {
                n179 = call <vilib>:"NT Read Number.vi"("Name"=w292) -> ("Numeric"=w291:dbl)  [unwired: 9 in, 1 out]
                n180 = local write "Test Slider"(w291) -> ()
                n181 = property on="Test Slider" class="Slide (strict)"("Visible"=TRUE, "Scale.Maximum"=100.0 ("Scale.Range:Maximum")) -> ()  [unwired: 2 in, 2 out]
                n182 = property on="Test Ring" class="Ring (strict)"("Visible"=FALSE) -> ()  [unwired: 2 in, 2 out]
              }
            }
          }
        }
        n183 = property on="Progress" class="Clust (strict)"("Visible"=FALSE) -> ()  [unwired: 2 in, 2 out]
      }
      event "Test Name": Mouse Enter {
        # "Populate the ring with the list of tests"
        n184 = event-data() -> ()  [unwired: 1 in, 1 out]
        n185 = call <vilib>:"NT Read String Array.vi"("Name"="TestMode/TestList") -> ("String Array"=w300:string[])  [unwired: 9 in, 1 out]
        n186 = Build Array (concatenate)("Select the test to run...", w300) -> (w299:string[])
        n187 = property on="Test Name" class="Ring (strict)"("Strings []"=w299) -> ()  [unwired: 2 in, 2 out]
      }
      event "Test Name": Value Change {
        w302 = FALSE ("Visible")
        # "Tell the robot the test name to run"
        n188 = event-data() -> ("NewVal"=w306:u16)  [unwired: 1 in]
        n189 = property on="Test Name" class="Ring (strict)"() -> ("Strings []"=w307:string[])  [unwired: 2 in, 2 out]
        n190 = local write "Progress"(T9 {"Test Progress"=0, "Test Progress Text"=""} ("Progress")) -> ()
        n191 = Index Array(array=w307, index=w306) -> (element=w305:string)
        n192 = call <vilib>:"NT Write String.vi"("String"=w305, "Name"="TestMode/TestName") -> ()  [unwired: 9 in, 1 out]
        n193 = property on="Progress" class="Clust (strict)"("Visible"=TRUE) -> ()  [unwired: 2 in, 2 out]
        n194 = property on="Motor" class="Clust (strict)"("Visible"=w302) -> ()  [unwired: 2 in, 2 out]
        n195 = property on="Test Slider" class="Slide (strict)"("Visible"=w302) -> ()  [unwired: 2 in, 2 out]
        n196 = property on="On/Off" class="Bool (strict)"("Visible"=w302) -> ()  [unwired: 2 in, 2 out]
        n197 = property on="Rev/Fwd" class="Clust (strict)"("Visible"=w302) -> ()  [unwired: 2 in, 2 out]
        n198 = property on="Test Ring" class="Ring (strict)"("Visible"=w302) -> ()  [unwired: 2 in, 2 out]
      }
      event "Listbox": Double Click {
        n199 = event-data() -> ("PlatMods.Shift"=w310:bool, "Row"=w312:i32)  [unwired: 1 in]
        n200 = case shown="True" w310 {
          tunnel: w312 -> [w316 _]
          tunnel: 1 -> [w315 _]
          frame False {
            n201 = property on="Listbox" class="LstBox (strict)"() -> ("Item Symbols"=w314:i32[])  [unwired: 2 in, 2 out]
            n202 = Replace Array Subset(array=w314, new element=w315, index=w316) -> (w313:i32[])
            n203 = property on="Listbox" class="LstBox (strict)"("Item Symbols"=w313) -> ()  [unwired: 2 in, 2 out]
          }
          frame True {
            w317 = 0 ("Top Row")
            n204 = property on="Listbox" class="LstBox (strict)"() -> ("Number of Rows"=w319:u32)  [unwired: 2 in, 2 out]
            n205 = Initialize Array(0, w319) -> (w318:i32[])
            n206 = property on="Listbox" class="LstBox (strict)"("Top Row"=w317, "Value"=w317, "Item Symbols"=w318) -> ()  [unwired: 2 in, 2 out]
          }
        }
      }
      event "Listbox": Key Down {
        n207 = event-data() -> ("VKey"=w323:T16)  [unwired: 1 in]
        n208 = case shown="\"Left\", \"Right\"" w323 {
          selector: w323 -> [w328 _]
          tunnel: eventvkey."Left" ("VKey") -> [w326 _]
          frame "Left", "Right" {
            n209 = Equal?(x=w326, y=w328) -> (x = y?=w327:bool)
            n210 = Select(t=0, s=w327, f=1) -> (s? t:f=w329:i32)
            n211 = property on="Listbox" class="LstBox (strict)"() -> ("Item Symbols"=w332:i32[])  [unwired: 2 in, 2 out]
            n212 = Replace Array Subset(array=w332, new element=w329, index="Listbox") -> (w331:i32[])
            n213 = property on="Listbox" class="LstBox (strict)"("Item Symbols"=w331) -> ()  [unwired: 2 in, 2 out]
          }
          frame Default {
          }
        }
      }
      event "DB Camera Config": Value Change {
        n214 = event-data() -> ("NewVal"=w336:bool)  [unwired: 1 in]
        n215 = case shown="False" w336 {
          tunnel: w335 -> [w345 _]
          tunnel: [w338 w356] -> w334
          tunnel: w333 -> [w337 w356]
          frame False {
            w352 = "Camera"
            w355 = FALSE ("Visible")
            n216 = local read "Camera Settings"() -> (w344:T2)
            n217 = Index Array(array=w345) -> (element=w348:cluster{string[]})  [unwired: 1 in]
            n218 = Unbundle(w344) -> ("Frame Rate"=w343:i32, "Compression"=w342:i32, "Size"=w346:u16)
            n219 = Unbundle(w348) -> (w347:string[])
            n220 = Index Array(array=w347, index=w346) -> (element=w341:string)
            n221 = call-poly <vilib>:"Write Key.vi"("section"=w352, "value"=w341, "key"="Size", "refnum"=w337) -> ("refnum out"=w354:T15)  [unwired: 2 in, 5 out]
            n222 = call-poly <vilib>:"Write Key.vi"("section"=w352, "value"=w343, "key"="FrameRate", "refnum"=w354) -> ("refnum out"=w353:T15)  [unwired: 1 in, 6 out]
            n223 = property on="Camera Settings" class="Clust (strict)"("Visible"=w355) -> ()  [unwired: 2 in, 2 out]
            n224 = local write "DB Camera Config"(w355) -> ()
            n225 = call-poly <vilib>:"Write Key.vi"("section"=w352, "value"=w342, "key"="Compression", "refnum"=w353) -> ("refnum out"=w339:T15)  [unwired: 1 in, 6 out]
            n226 = call <vilib>:"Close Config Data.vi"("refnum"=w339) -> ("file path"=w340:path)  [unwired: 2 in, 8 out]
            n227 = call <vilib>:"Open Config Data.vi"("configuration file path"=w340) -> ("refnum"=w338:T15)  [unwired: 8 in, 2 out]
          }
          frame True {
            n228 = property on="Camera Settings" class="Clust (strict)"("Visible"=TRUE) -> ()  [unwired: 2 in, 2 out]
          }
        }
      }
      event "Camera Settings": Value Change {
        n229 = event-data() -> ("NewVal"=w369:T2)  [unwired: 1 in]
        n230 = Index Array(array=w365) -> (element=w364:cluster{string[]})  [unwired: 1 in]
        n231 = Unbundle(w369) -> ("Frame Rate"=w360:i32, "Compression"=w359:i32, "Size"=w362:u16)
        n232 = Unbundle(w364) -> (w363:string[])
        n233 = Index Array(array=w363, index=w362) -> (element=w361:string)
        n234 = Format Into String(format string="%s   %dfps   %d%%", w361, w360, w359) -> (resulting string=w366:string)  [unwired: 2 in, 1 out]
        n235 = Build Array(w366) -> (w367:string[])
        n236 = property on="DB Camera Config" class="Bool (strict)"("Strings [4]"=w367) -> ()  [unwired: 2 in, 2 out]
      }
      event "Motor.Enable": Value Change {
        n237 = event-data() -> ("NewVal"=w375:bool)  [unwired: 1 in]
        n238 = Unbundle("Motor") -> ("Value"=w374:dbl)  [unwired: 1 out]
        n239 = Select(t=w374, s=w375, f=0.0) -> (s? t:f=w372:dbl)
        n240 = call <vilib>:"NT Write Number.vi"("Numeric"=w372, "Name"=w371) -> ()  [unwired: 9 in, 1 out]
      }
      event "Test Slider": Value Change {
        n241 = event-data() -> ("NewVal"=w378:dbl)  [unwired: 1 in]
        n242 = call <vilib>:"NT Write Number.vi"("Numeric"=w378, "Name"=w379) -> ()  [unwired: 9 in, 1 out]
      }
      event "On/Off": Value Change {
        n243 = event-data() -> ("NewVal"=w383:bool)  [unwired: 1 in]
        n244 = Boolean To (0,1)(Boolean=w383) -> (0, 1=w382:i16)
        n245 = call <vilib>:"NT Write Number.vi"("Numeric"=w382, "Name"=w381) -> ()  [unwired: 9 in, 1 out]
      }
      event "Rev/Fwd": Value Change {
        n246 = event-data() -> ("NewVal.Forward"=w391:bool, "NewVal.Reverse"=w390:bool)  [unwired: 1 in]
        n247 = Boolean To (0,1)(Boolean=w391) -> (0, 1=w387:i16)
        n248 = Boolean To (0,1)(Boolean=w390) -> (0, 1=w389:i16)
        n249 = Negate(x=w389) -> (-x=w388:i16)
        n250 = Add(x=w387, y=w388) -> (x+y=w386:i16)
        n251 = call <vilib>:"NT Write Number.vi"("Numeric"=w386, "Name"=w385) -> ()  [unwired: 9 in, 1 out]
      }
      event "Test Ring": Value Change {
        n252 = event-data() -> ("NewVal"=w395:u16)  [unwired: 1 in]
        n253 = property on="Test Ring" class="Ring (strict)"() -> ("Strings []"=w396:string[])  [unwired: 2 in, 2 out]
        n254 = Index Array(array=w396, index=w395) -> (element=w394:string)
        n255 = call <vilib>:"NT Write String.vi"("String"=w394, "Name"=w393) -> ()  [unwired: 9 in, 1 out]
      }
      event "Rec Mode": Value Change {
        # "Update globals for recording mode and path to read log from.\nClear when logging and let NetworkTables set path for vision to\nuse."
        n256 = event-data() -> ("NewVal"=w406:enum32{"Stop", "Record", "Playback"})  [unwired: 1 in]
        n257 = global write "WPI_DashboardLogging Global.vi" "Logging Filename"(path "") -> ()
        n258 = case shown="\"Stop\", \"Record\"" w406 {
          tunnel: w405 -> [_ w408 w416]
          tunnel: [_ _ w415] -> w402
          tunnel: [_ _ w414] -> _
          tunnel: w400 -> [_ _ w412]
          tunnel: cluster{i32, i32} {-250, 170} -> [_ _ w411]
          tunnel: [_ _ T17 {"Image Size"=TRUE, "Image Type"=TRUE, "Pixel Value"=TRUE, "ROI Information"=TRUE, "Zoom Factor"=FALSE} ("Image Information Shown:All Elements")] -> w398
          tunnel: [_ _ TRUE ("Zoom Factor")] -> w397
          frame Default {
          }
          frame "Stop", "Record" {
            # "Place Window too"
            n259 = invoke class="VI" method="FP.Close"(reference=w408) -> (reference out=w407:refnum<vi>)  [unwired: 2 in, 2 out]
            n260 = invoke class="VI" method="Abort VI"(reference=w407) -> ()  [unwired: 2 in, 3 out]
          }
          frame "Playback" {
            n261 = call "Open Playback Panel.vi"("Offset"=w411, "DB VI Ref"=w412, "Playback in"=w416) -> ("Playback out"=w413:refnum<vi>)  [unwired: 8 in]
            n262 = register-events(w413) -> (reference out=w415:refnum<event-registration>, error out=w414:errorcluster)  [unwired: 2 in]
          }
        }
        n263 = global write "WPI_DashboardLogging Global.vi" "Recording"(w406) -> ()
        n264 = property on="Camera Image" class="ImageControl"("Image Information Shown"=w398, "Image Information Visible"=w397) -> ()  [unwired: 2 in, 2 out]
        n265 = call <vilib>:"WPI_DashboardNT Log FieldName Cache.vi"("Operation"=enum16{"Lookup/Add", "Index", "Clear"}."Clear") -> ()  [unwired: 8 in, 3 out]
      }
      event Panel Close {
        w417 = enum32{"Stop", "Record", "Playback"}."Stop" ("Rec Mode")
        n266 = event-data() -> ()  [unwired: 1 in, 4 out]
        n267 = local write "Rec Mode"(w417) -> ()
        n268 = global write "WPI_DashboardLogging Global.vi" "Recording"(w417) -> ()
      }
      event Panel Close {
        # "Abort playback window and ourself"
        n269 = event-data() -> ()  [unwired: 1 in, 4 out]
        n270 = invoke class="VI" method="FP.Close"(reference=w422) -> (reference out=w421:refnum<vi>)  [unwired: 2 in, 2 out]
        n271 = invoke class="VI" method="Abort VI"(reference=w421) -> (error out=w420:errorcluster)  [unwired: 2 in, 2 out]
        n272 = invoke class="VI" method="Abort VI"(error in=w420) -> ()  [unwired: 2 in, 3 out]
      }
    }
  }
  n273 = property on="On/Off" class="Bool (strict)"("Visible"=w25) -> ()  [unwired: 2 in, 2 out]
  n274 = property on="Motor" class="Clust (strict)"("Visible"=w25) -> ()  [unwired: 2 in, 2 out]
  n275 = property on="Progress" class="Clust (strict)"("Visible"=w25) -> ()  [unwired: 2 in, 2 out]
  n276 = property on="Test Ring" class="Ring (strict)"("Visible"=w25) -> ()  [unwired: 2 in, 2 out]
  n277 = property on="Rev/Fwd" class="Clust (strict)"("Visible"=w25) -> ()  [unwired: 2 in, 2 out]
  n278 = property on="Camera Settings" class="Clust (strict)"("Visible"=w25) -> ()  [unwired: 2 in, 2 out]
  n279 = local write "DB Camera Config"(w25) -> ()
  n280 = global write "WPI_DashboardLogging Global.vi" "Recording"(w8) -> ()
  n281 = local write "Rec Mode"(w8) -> ()
